vi "FindTarget.vi"(0 "Image In":T2, 7 "error in":errorcluster) -> (20 "Image Out":T2, 21 "Matches (Pattern Matching 1)":T1(array[cluster]) {"Bounding Box"."y" format="%.2f"; "Bounding Box"."x" format="%.2f"; "Position"."y" format="%.2f"; "Position"."x" format="%.2f"; "Score" format="%.2f"; "Scale" format="%.2f"; "Angle" format="%.2f"}, 22 "Calibrated Matches (Pattern Matching 1)":T1(array[cluster]) {"Bounding Box"."y" format="%.2f"; "Bounding Box"."x" format="%.2f"; "Position"."y" format="%.2f"; "Position"."x" format="%.2f"; "Score" format="%.2f"; "Scale" format="%.2f"; "Angle" format="%.2f"}, 23 "Number of Matches (Pattern Matching 1)":i32, 27 "error out":errorcluster)   [LabVIEW 2017]
uses:
  <vilib>/vision/Image Controls.llb/IMAQ Image.ctl
  <vilib>/vision/NI_Vision_Development_Module.lvlib
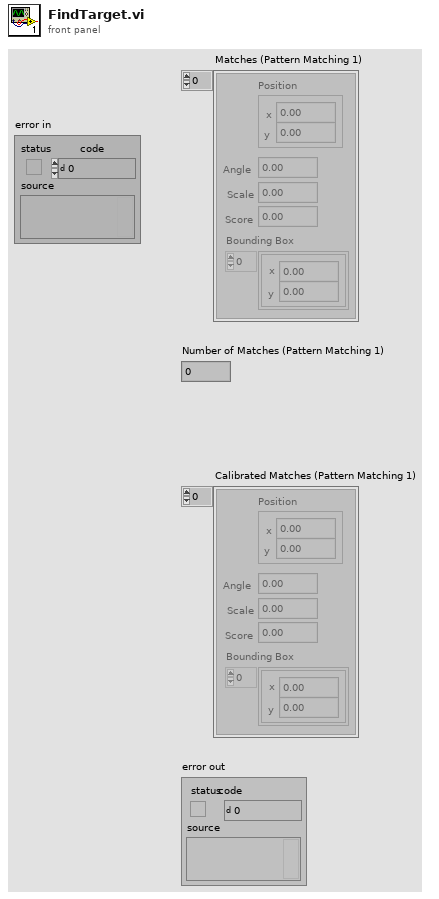
[diagram p1: front panel]
types:
  T1 = cluster{"Position":cluster{"x":sgl, "y":sgl}, "Angle":sgl, "Scale":sgl, "Score":sgl, "Bounding Box":cluster{"x":sgl, "y":sgl}[]}[]
  T2 = typedef "IMAQ Image.ctl" = refnum<image>
  T3 = cluster{"Number of Matches Requested":i32, "Minimum Match Score":sgl, "Angle Ranges":cluster{"Start Angle":sgl, "End Angle":sgl}[]}
  T4 = cluster{"Global Rectangle":i32[], "Contours":cluster{"ID":enum32{"External", "Internal"}, "Type":u32, "Coordinates":i32[]}[]}
  T5 = typedef "Image Type" = u32
  T6 = cluster{"Brightness":sgl, "Contrast":sgl, "Gamma":sgl}
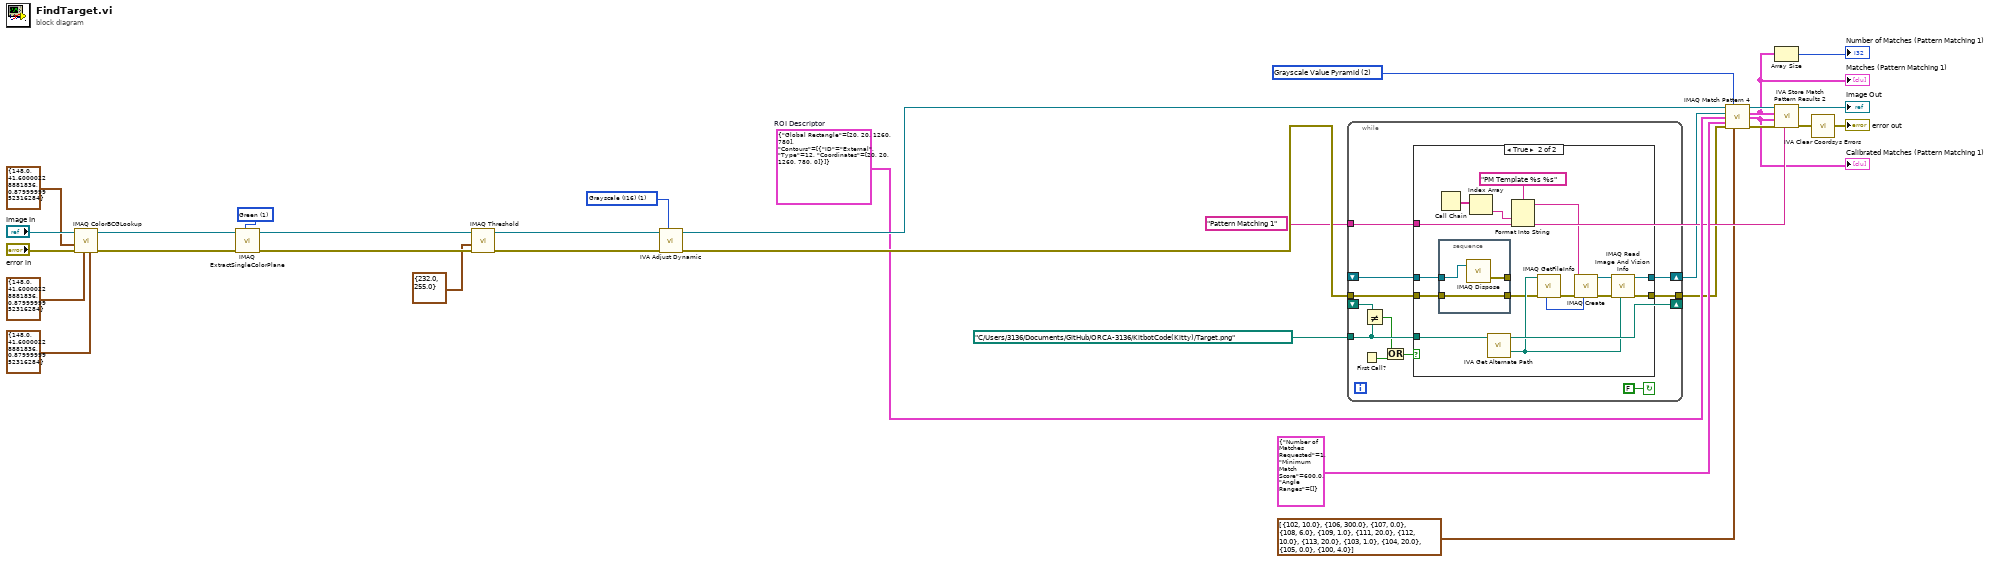
[diagram p0: block diagram]
diagram:
  w12 = 2 items=["All", "Low Discrepancy Sampling", "Grayscale Value Pyramid", "Gradients Pyramid"] ("Algorithm")
  w8 = "Pattern Matching 1" ("Step Name")
  w11 = T4 {"Global Rectangle"=[20, 20, 1260, 780], "Contours"=[{"ID"=enum."External", "Type"=12, "Coordinates"=[20, 20, 1260, 780, 0]}]}  # ROI Descriptor
  w18 = T5 1 items=["Grayscale (U8)", "Grayscale (I16)", "Grayscale (SGL)", "Complex (CSG)", "RGB (U32)", "HSL (U32)", "RGB (U64)", "Grayscale (U16)"] ("Image Type")
  w26 = 1 items=["Red", "Green", "Blue", "Hue", "Saturation", "Luminance", "Value", "Intensity"] ("Color Plane")
  n1 = call "IMAQ ColorBCGLookup"("Blue BCG Values"=T6 {"Brightness"=148.0, "Contrast"=41.600002, "Gamma"=0.88}, "Green BCG Values"=T6 {"Brightness"=148.0, "Contrast"=41.600002, "Gamma"=0.88}, "error in (no error)"="error in", "Red BCG Values"=T6 {"Brightness"=148.0, "Contrast"=41.600002, "Gamma"=0.88}, "Image Src"="Image In") -> ("error out"=w30:errorcluster, "Image Dst Out"=w25:T2)  [unwired: 2 in, 3 out]
  n2 = call "IMAQ ExtractSingleColorPlane"("Color Plane"=w26, "error in (no error)"=w30, "Image Src"=w25) -> ("error out"=w24:errorcluster, "Image Dst Out"=w22:T2)  [unwired: 1 in, 6 out]
  n3 = call "IMAQ Threshold"("error in (no error)"=w24, "Range"=cluster{"Lower value":sgl, "Upper value":sgl} {"Lower value"=232.0, "Upper value"=255.0}, "Image Src"=w22) -> ("error out"=w21:errorcluster, "Image Dst Out"=w20:T2)  [unwired: 3 in, 4 out]
  n4 = call <vilib>:"IVA Adjust Dynamic.vi"("Image Type"=w18, "error in (no error)"=w21, "Image Src"=w20) -> ("error out"=w19:errorcluster, "Image Out"=w16:T2)  [unwired: 7 out]
  n5 = while {
    shift-right: [w43] -> w5
    shift-left: _ -> [w42]
    tunnel: [w40] -> w4
    tunnel: w19 -> [w39]
    tunnel: path "C:/Users/3136/Documents/GitHub/ORCA-3136/KitbotCode(Kitty)/Target.png" ("Template File Path") -> [w36]
    tunnel: w8 -> [w38]
    shift-right: [w36] -> _
    shift-left: _ -> [w37]
    stop <- FALSE continue-if-true
    n6 = First Call?() -> (First Call?: T/F=w35:bool)
    n7 = Not Equal?(x=w37, y=w36) -> (x != y?=w34:bool)
    n8 = Or(x=w34, y=w35) -> (x .or. y?=w33:bool)
    n9 = case shown="True" w33 {
      tunnel: [w45 w59] -> w43
      tunnel: w42 -> [w45 w51]
      tunnel: [w44 w56] -> w40
      tunnel: w39 -> [w44 w50]
      tunnel: w36 -> [_ w52]
      tunnel: w38 -> [_ w53]
      frame False {
      }
      frame True {
        n10 = stacked-sequence {
          tunnel: w51 -> [w64]
          tunnel: w50 -> [w63]
          tunnel: [w63] -> w46
          tunnel: [w62] -> _
          frame #0 {
            n11 = call "IMAQ Dispose"("Image"=w64) -> ("error out"=w62:errorcluster)  [unwired: 2 in, 3 out]
          }
        }
        n12 = Call Chain() -> (call chain=w55:string[])
        n13 = Index Array(array=w55) -> (element=w54:string)  [unwired: 1 in]
        n14 = call <vilib>:"IVA Get Alternate Path.vi"("Path In"=w52) -> ("Path Out"=w48:path)  [unwired: 10 out]
        n15 = Format Into String(format string="PM Template %s %s" ("Image Name"), w54, w53) -> (resulting string=w61:string)  [unwired: 2 in, 1 out]
        n16 = call "IMAQ GetFileInfo"("error in (no error)"=w46, "File Path"=w48) -> ("error out"=w47:errorcluster, "Image Type"=w49:T5)  [unwired: 3 in, 5 out]
        n17 = call "IMAQ Create"("Image Name"=w61, "Image Type"=w49, "error in (no error)"=w47) -> ("New Image"=w58:T2, "error out"=w57:errorcluster)  [unwired: 1 in, 1 out]
        n18 = call "IMAQ Read Image And Vision Info"("File Path"=w48, "error in (no error)"=w57, "Image"=w58) -> ("error out"=w56:errorcluster, "Image Out"=w59:T2)  [unwired: 1 in, 6 out]
      }
    }
  }
  n19 = call "IMAQ Match Pattern 4"("Image"=w16, "Algorithm"=w12, "Template Image"=w5, "ROI Descriptor"=w11, "Parameters"=T3 {"Number of Matches Requested"=1, "Minimum Match Score"=600.0, "Angle Ranges"=[]}, "error in (no error)"=w4, "Advanced Options"=cluster{"Item":u16, "Value":dbl}[] [{"Item"=102, "Value"=10.0}, {"Item"=106, "Value"=300.0}, {"Item"=107, "Value"=0.0}, {"Item"=108, "Value"=6.0}, {"Item"=109, "Value"=1.0}, {"Item"=111, "Value"=20.0}, {"Item"=112, "Value"=10.0}, {"Item"=113, "Value"=20.0}, {"Item"=103, "Value"=1.0}, {"Item"=104, "Value"=20.0}, {"Item"=105, "Value"=0.0}, {"Item"=100, "Value"=4.0}]) -> ("Image (duplicate)"=w13:T2, "Matches (pixel)"=w7:T1, "Matches (real-world)"=w6:T1, "error out"=w14:errorcluster)  [unwired: 4 in, 1 out]
  "Matches (Pattern Matching 1)" <- w7
  "Calibrated Matches (Pattern Matching 1)" <- w6
  n20 = Array Size(array=w7) -> (size(s)=→"Number of Matches (Pattern Matching 1)":i32)
  n21 = call <vilib>:"IVA Store Match Pattern Results 2.vi"("Step Name"=w8, "error in (no error)"=w14, "Matches (real-world)"=w6, "Matches (pixel)"=w7, "Image in"=w13) -> ("error out"=w3:errorcluster, "Image dup"=→"Image Out":T2)  [unwired: 1 in, 4 out]
  n22 = call <vilib>:"IVA Clear Coordsys Errors.vi"("error in (no error)"=w3) -> ("error out"=→"error out":errorcluster)  [unwired: 10 in]
